vi "MGI Threshold 1D Array Extended.vi"(1 "Start Index (0)":i32, 2 "Threshold Y":dbl, 3 "Y Value[]":dbl[](array[numeric])) -> (0 "Extended Fractional Index":dbl)   [LabVIEW 2019]
doc: "Extended version of threshold which can produce fractional indices outside of the array limits. Linear extension based on the first or last two array elements is used for out of range values.\n\nAuthored by David A. Moore\nsupport@mooregoodideas.com\nwww.mooregoodideas.com\n\nCopyright (c) 2010, Moore Good Ideas, Inc.\n\nAll rights reserved.\n\nRedistribution and use in source and binary forms, with or without modification, are permitted provided that the following conditions are met:\n\n * Redistributions of source code must retain the above copyright notice, this list of conditions and the following disclaimer.\n * Redistributions in binary form must reproduce the above copyright notice, this list of conditions and the following disclaimer in the documentation and/or other materials provided with the distribution.\n * Neither the name of Moore Good Ideas, Inc. nor the names of its contributors may be used to endorse or promote products derived from this software without specific prior written permission.\n\nTHIS SOFTWARE IS PROVIDED BY THE COPYRIGHT HOLDERS AND CONTRIBUTORS \"AS IS\" AND ANY EXPRESS OR IMPLIED WARRANTIES, INCLUDING, BUT NOT LIMITED TO, THE IMPLIED WARRANTIES OF MERCHANTABILITY AND FITNESS FOR A PARTICULAR PURPOSE ARE DISCLAIMED. IN NO EVENT SHALL THE COPYRIGHT OWNER OR CONTRIBUTORS BE LIABLE FOR ANY DIRECT, INDIRECT, INCIDENTAL, SPECIAL, EXEMPLARY, OR CONSEQUENTIAL DAMAGES (INCLUDING, BUT NOT LIMITED TO, PROCUREMENT OF SUBSTITUTE GOODS OR SERVICES; LOSS OF USE, DATA, OR PROFITS; OR BUSINESS INTERRUPTION) HOWEVER CAUSED AND ON ANY THEORY OF LIABILITY, WHETHER IN CONTRACT, STRICT LIABILITY, OR TORT (INCLUDING NEGLIGENCE OR OTHERWISE) ARISING IN ANY WAY OUT OF THE USE OF THIS SOFTWARE, EVEN IF ADVISED OF THE POSSIBILITY OF SUCH DAMAGE."
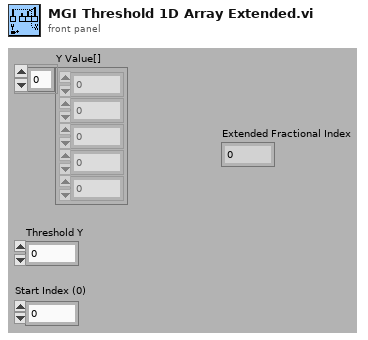
[diagram p1: front panel]
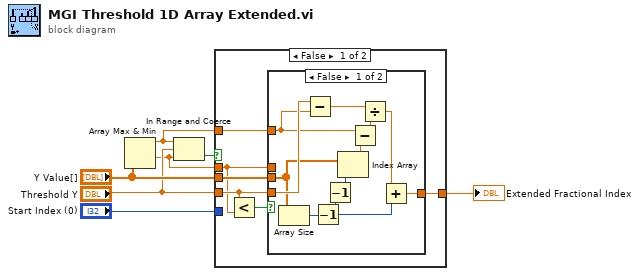
[diagram p0: block diagram]
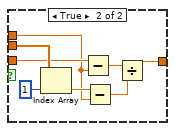
[diagram p2: hidden frame]
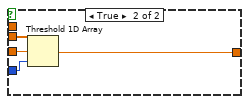
[diagram p3: hidden frame]
diagram:
  n1 = Array Max & Min(array="Y Value[]") -> (max value=w3:dbl, min value=w2:dbl)  [unwired: 2 out]
  n2 = In Range and Coerce(upper limit=w3, x="Threshold Y", lower limit=w2) -> (In Range?=w4:bool)  [unwired: 1 out]
  n3 = case shown="False" w4 {
    tunnel: [w9 w36] -> w7
    tunnel: "Y Value[]" -> [w12 w35]
    tunnel: "Threshold Y" -> [w11 w34]
    tunnel: w3 -> [w8 _]
    tunnel: w2 -> [w10 _]
    tunnel: "Start Index (0)" -> [_ w33]
    frame False {
      n4 = Less?(x=w11, y=w10) -> (x < y?=w13:bool)
      n5 = case shown="False" w13 {
        tunnel: w12 -> [w19 w32]
        tunnel: w11 -> [w24 w30]
        tunnel: w10 -> [_ w28]
        tunnel: [w16 w25] -> w9
        tunnel: w8 -> [w23 _]
        frame False {
          n6 = Array Size(array=w19) -> (size(s)=w18:i32)
          n7 = Subtract(x=w24, y=w23) -> (x-y=w20:dbl)
          n8 = Decrement(x=w18) -> (x-1=w14:i32)
          n9 = Decrement(x=w14) -> (x-1=w15:i32)
          n10 = Index Array(array=w19, index=w15) -> (element=w22:dbl)
          n11 = Subtract(x=w23, y=w22) -> (x-y=w21:dbl)
          n12 = Divide(x=w20, y=w21) -> (x/y=w17:dbl)
          n13 = Add(x=w17, y=w14) -> (x+y=w16:dbl)
        }
        frame True {
          n14 = Index Array(array=w32, index=1) -> (element=w29:dbl)
          n15 = Subtract(x=w30, y=w28) -> (x-y=w27:dbl)
          n16 = Subtract(x=w29, y=w28) -> (x-y=w26:dbl)
          n17 = Divide(x=w27, y=w26) -> (x/y=w25:dbl)
        }
      }
    }
    frame True {
      n18 = Threshold 1D Array(1:w33, 2:w34, 3:w35) -> (0:w36:dbl)
    }
  }
  "Extended Fractional Index" <- w7
